vi "STM主程序（队列输入）-测试3.vi"() -> ()   [LabVIEW 2015]
uses:
  <vilib>/NI/STM/TCP/Write Meta Data (TCP Ref).vi
  <vilib>/NI/STM/NI STM.lvlib
  <vilib>/NI/STM/SubVIs/MetaDataElement.ctl
  <vilib>/NI/STM/TCP/Get Connection Reference (TCP).vi
  <vilib>/NI/STM/TCP/TCP Read Options.ctl
  <vilib>/NI/STM/TCP/Read Message (TCP).vi
  <vilib>/NI/STM/TCP/Write Message (TCP).vi
panel:
  in  "阈值等级":i32=4
  in  "Stop (F)":bool
  in  "关闭程序":bool
  out "触发":bool
  in  "?":bool
  out "自动后退":bool
  in  "?":bool
  out "自动前进":bool
  in  "?":bool
  out "步进距离":u16
  out "error  out":errorcluster
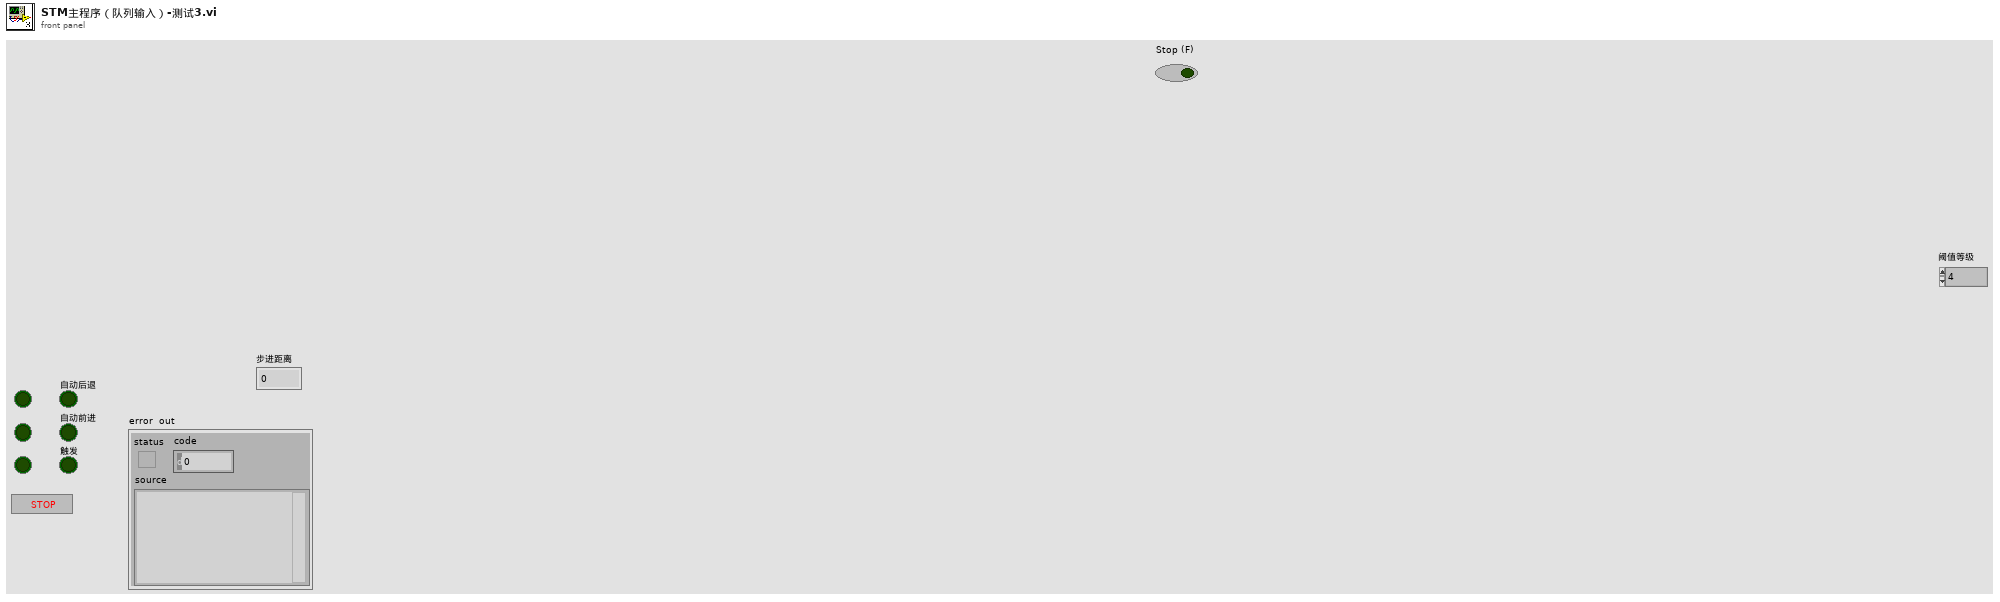
[diagram p1: front panel]
types:
  T1 = typedef "NI STM.lvlib/MetaDataElement.ctl" = string
  T2 = typedef "NI STM.lvlib/TCP Connection Info.ctl" = cluster{"connection ID":refnum<k5>, "meta data":T1[]}
  T3 = cluster{"图像数据":refnum<queue>, "队列输出":refnum<queue>}
  T4 = typedef "IMAQ Image.ctl" = refnum<image>
  T5 = cluster{"滤波":T4, "边缘检测":T4, "untitled":T4, "3D view":T4, "灰度图像":T4}
  T6 = cluster{"周长":dbl, "面积":dbl, "3D":u8[], "灰度图像":T4, "3D view":T4, "滤波":T4, "边缘检测":T4, "3D图像":T4, "质心坐标X":sgl, "质心坐标Y":sgl, "第一点y值，x=0":dbl, "第二点y值，x=639":dbl, "第一点x值，y=0":dbl, "第二点x值，y=479":dbl, "短轴半径um":dbl, "长轴半径um":dbl, "长轴长度":dbl, "短轴长度":dbl, "短轴原曲线":dbl[], "长轴拟合":dbl[], "纵轴拟合":dbl[], "横轴拟合":dbl[], "长轴原曲线":dbl[], "纵轴原曲线":dbl[], "横轴原曲线":dbl[], "短轴拟合":dbl[], "位置":dbl, "触发":bool, "初始化后退":bool, "初始化前进":bool}
  T7 = typedef "NI STM.lvlib/TCP Read Options.ctl" = cluster{"ignore timeout error":bool, "timeout ms (1000)":i32}
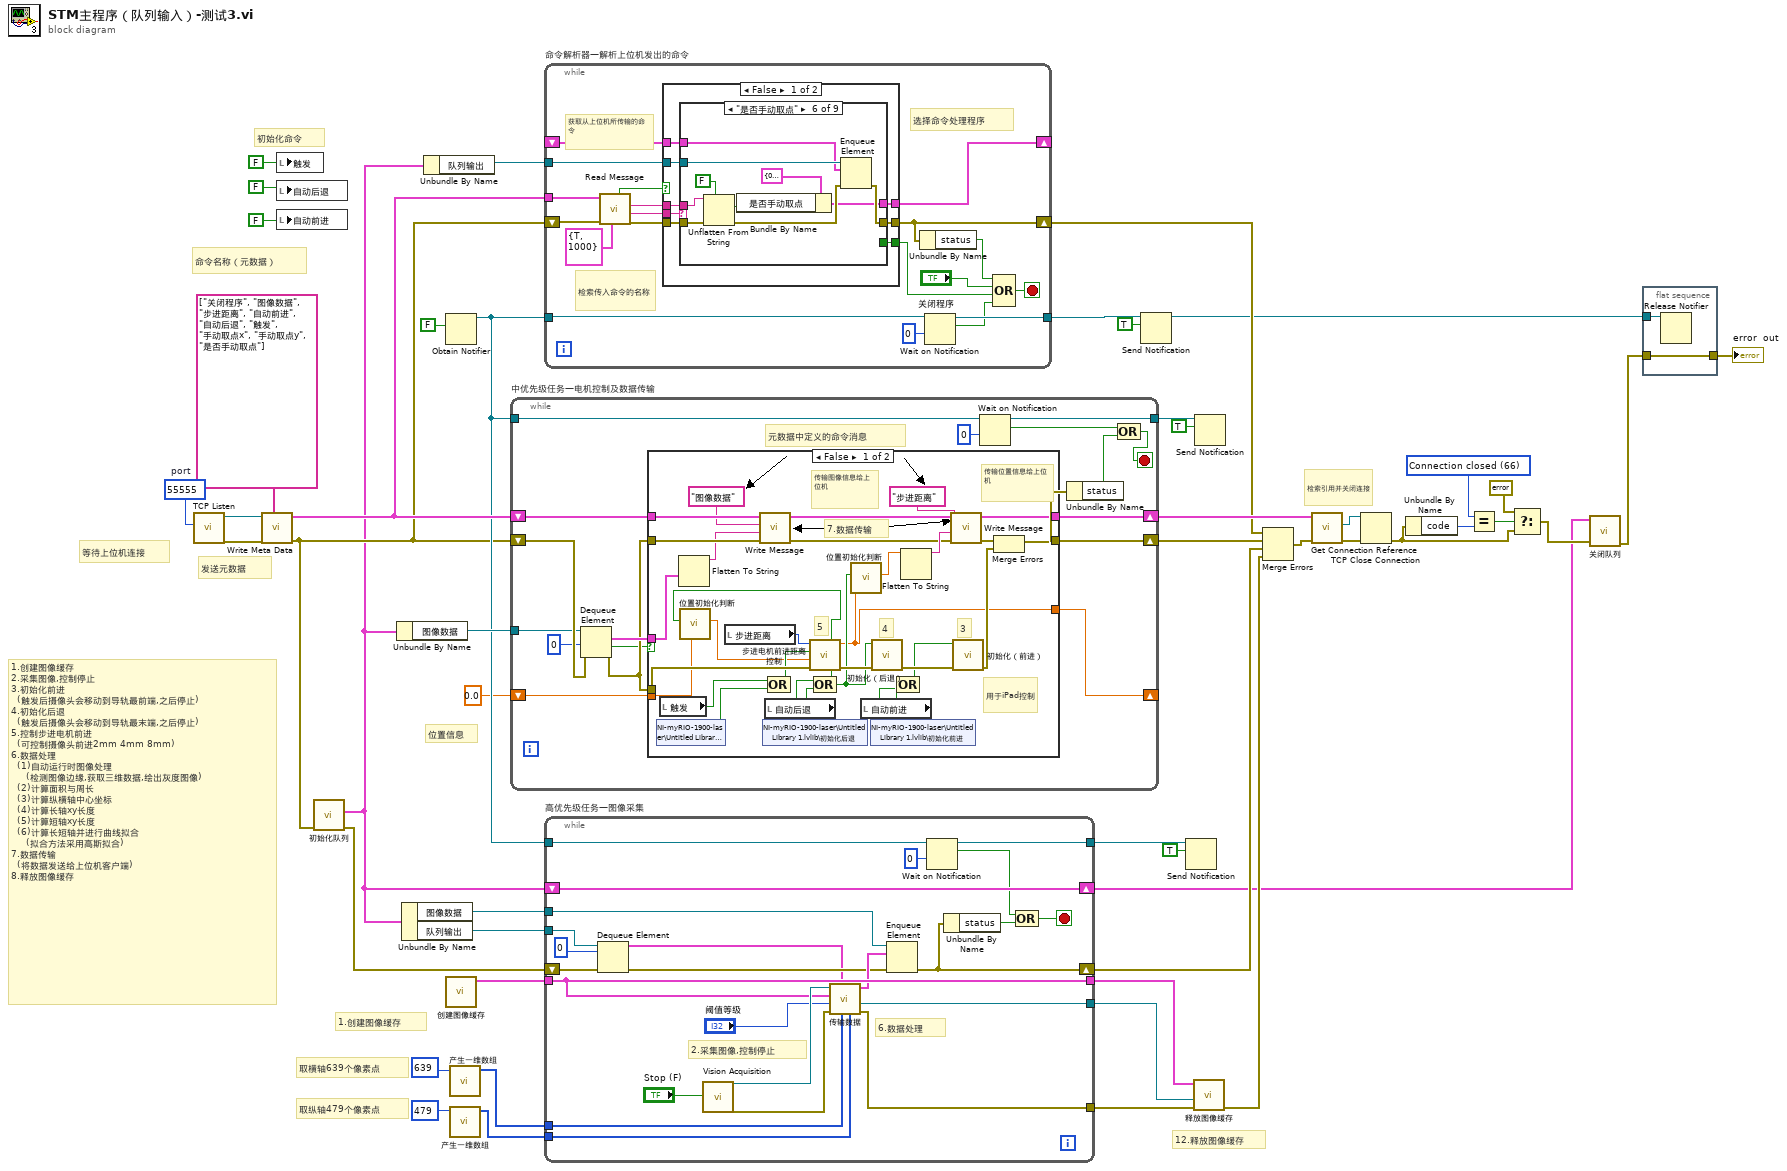
[diagram p0: block diagram]
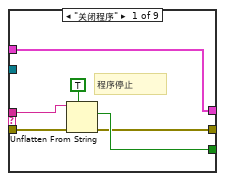
[diagram p3: hidden frame]
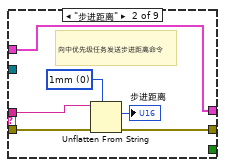
[diagram p4: hidden frame]
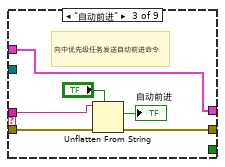
[diagram p5: hidden frame]
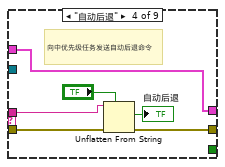
[diagram p6: hidden frame]
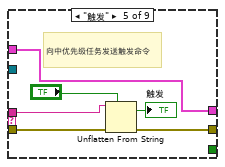
[diagram p7: hidden frame]
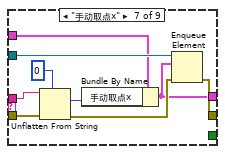
[diagram p8: hidden frame]
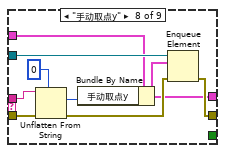
[diagram p9: hidden frame]
diagram:
  w24 = 66 items=["No Error", "Argument Error", "Memory Full", "Out of Zone", "End of File", "File Already Open", "Generic File IO Error", "File Not Found", "File Permission Error", "Disk Full", "Duplicate Path", "Too Many Files Open", "Not Enabled", "Resource File Not Found", "Cannot Add Resource", "Resource Not Found", "Image Not Found", "Image Memory Error", "Pen Does Not Exist", "Config Bad Type", "Config Token Not Found", "Config Parse Error", "Config Memory Error", "Bad External Code Format", "Bad External Code Offset", "External Code Not Present", "Null Window", "Destroy Window Mixup", "Null Menu", "Print Aborted", "Bad Print Record", "Print Driver Error", "Windows Error During Print", "Memory Error During Print", "Print Dialog Error", "Generic Print Error", "Invalid Device Refnum", "Device Not Found", "Device Parameter Error", "Device Unit Error", "Can't Open Device", "Device Call Aborted", "Generic Error", "Cancelled By User", "Object ID Too Low", "Object ID Too High", "Object Not In Heap", "Unknown Heap", "Bad DefProc ID", "DefProc Not In Table", "Message Out Of Range", "Null Method", "Unknown Message", "Manager Call Not Supported", "Bad address", "Connection In progress", "Connection timed out", "Connection is already in progress", "Network attribute not supported", "Network error", "Address in use", "System out of memory", "Connection aborted", "Connection refused", "Connection is not connected", "Connection is already connected", "Connection closed", "Initialize error (interapplication manager)", "Bad occurrence", "Wait on unbound occurrence handler", "Occurrence queue overflow", "Bad path", "Semaphore not signaled", "Unrecognized type (interapplication manager)"] ("1st Error to Convert")
  w50 = u16 55555  # port
  # "位置信息"
  # "初始化命令"
  # "等待上位机连接"
  # "发送元数据"
  # "检索引用并关闭连接"
  # "命令名称（元数据）"
  # "1.创建图像缓存"
  # "1.创建图像缓存\n2.采集图像,控制停止\n3.初始化前进\n  (触发后摄像头会移动到导轨最前端,之后停止)\n4.初始化后退\n  (触发后摄像头会移动到导轨最末端,之后停止)\n5.控制步进电机前进\n  (可控制摄像头前进2mm 4mm 8mm)\n6.数据处理\n  (1)自动运行时图像处理\n     (检测图像边缘,获取三维数据,绘出灰度图像)\n  (2)计算面积与周长\n  (3)计算纵横轴中心坐标\n  (4)计算长轴xy长度\n  (5)计算短轴xy长度\n  (6)计算长短轴并进行曲线拟合\n     (拟合方法采用高斯拟合) \n7.数据传输 \n  (将数据发送给上位机客户端) \n8.释放图像缓存"
  # "取纵轴479个像素点"
  # "取横轴639个像素点"
  # "12.释放图像缓存"
  n1 = call <vilib>:"TCP Listen.vi"("port"=w50) -> ("error out"=w48:errorcluster, "connection ID"=w49:refnum<k5>)  [unwired: 3 in, 6 out]
  n2 = call-poly "Write Meta Data.vi"("meta data"=T1[] ["关闭程序", "图像数据", "步进距离", "自动前进", "自动后退", "触发", "手动取点x", "手动取点y", "是否手动取点"] ("Meta data"), "error in"=w48, "connection ID"=w49) -> ("error out"=w21:errorcluster, "connection info out"=w47:T2)  [unwired: 2 in, 5 out]
  n3 = local write "触发"(FALSE) -> ()
  n4 = local write "自动后退"(FALSE) -> ()
  n5 = local write "自动前进"(FALSE) -> ()
  n6 = call "初始化队列.vi"("error in (no error)"=w21) -> ("error out"=w20:errorcluster, "输出簇"=w3:T3)  [unwired: 9 in]
  n7 = Unbundle By Name(w3) -> ("图像数据"=w46:refnum<queue>)
  n8 = Unbundle By Name(w3) -> ("图像数据"=w45:refnum<queue>, "队列输出"=w1:refnum<queue>)
  n9 = Unbundle By Name(w3) -> ("队列输出"=w2:refnum<queue>)
  n10 = Obtain Notifier(notification data type=FALSE) -> (notifier out=w31:refnum<notifier>)  [unwired: 3 in, 2 out]
  n11 = call "创建图像缓存.vi"() -> ("簇"=w19:T5)  [unwired: 11 in]
  n12 = call "产生一维数组.vi"("Numeric"=639) -> ("Array"=w10:i32[])  [unwired: 10 in]
  n13 = call "产生一维数组.vi"("Numeric"=479) -> ("Array"=w9:i32[])  [unwired: 10 in]
  n14 = while "中优先级任务—电机控制及数据传输" {
    tunnel: w46 -> [w58]
    shift-right: [w60] -> w41
    shift-left: w21 -> [w64]
    shift-right: [w66] -> w44
    shift-left: w47 -> [w67]
    tunnel: w31 -> [w61]
    tunnel: [w59] -> w32
    shift-right: [w56] -> _
    shift-left: 0.0 ("x") -> [w57]
    stop <- w51 stop-if-true
    # "元数据中定义的命令消息"
    n15 = Dequeue Element(queue=w58, timeout in ms (-1)=0, error in (no error)=w64) -> (element=w65:T6, timed out?=w54:bool, error out=w55:errorcluster)  [unwired: 1 out]
    n16 = case shown="False" w54 {
      tunnel: w67 -> [w97 w100]
      tunnel: w55 -> [w96 w99]
      tunnel: [w89 w100] -> w66
      tunnel: [w83 w99] -> w60
      tunnel: w65 -> [w81 _]
      tunnel: w57 -> [w72 w98]
      tunnel: [w69 w98] -> w56
      tunnel: w55 -> [w82 _]
      frame False {
        # "传输图像信息给上位机"
        # "用于iPad控制"
        # "传输位置信息给上位机"
        # "7.数据传输"
        # "3"
        # "4"
        # "5"
        n17 = shared-variable "NI-myRIO-1900-laser\\Untitled Library 1.lvlib\\触发"() -> (w79:bool)  [unwired: 1 in, 1 out]
        n18 = local read "触发"() -> (w80:bool)
        n19 = Flatten To String(anything=w81) -> (data string=w94:string)  [unwired: 1 in, 4 out]
        n20 = local read "步进距离"() -> (w88:u16)
        n21 = call-poly "Write Message.vi"("error in"=w96, "data"=w94, "name"="图像数据" ("Name"), "connection info in"=w97) -> ("error out"=w90:errorcluster, "connection info out"=w91:T2)  [unwired: 1 in, 5 out]
        n22 = shared-variable "NI-myRIO-1900-laser\\Untitled Library 1.lvlib\\初始化后退"() -> (w76:bool)  [unwired: 1 in, 1 out]
        n23 = local read "自动后退"() -> (w77:bool)
        n24 = Compound Arithmetic op=OR(w80, w79) -> (w78:bool)
        n25 = Compound Arithmetic op=OR(w77, w76) -> (w70:bool)
        n26 = call "位置初始化判断.vi"("位置初始化"=w72, "是否后退"=w70) -> ("位置判断"=w71:dbl)  [unwired: 9 in]
        n27 = call "步进电机前进距离控制.vi"("error in"=w82, "初始化位置"=w71, "触发"=w78, "枚举"=w88) -> ("error out"=w87:errorcluster, "位置"=w69:dbl)  [unwired: 6 in]
        n28 = call "位置初始化判断.vi"("位置初始化"=w69, "是否后退"=w70) -> ("位置判断"=w68:dbl)  [unwired: 9 in]
        n29 = local read "自动前进"() -> (w75:bool)
        n30 = shared-variable "NI-myRIO-1900-laser\\Untitled Library 1.lvlib\\初始化前进"() -> (w74:bool)  [unwired: 1 in, 1 out]
        n31 = call "初始化（后退）.vi"("error in"=w87, "初始化"=w70) -> ("error out"=w86:errorcluster)  [unwired: 9 in]
        n32 = Compound Arithmetic op=OR(w75, w74) -> (w73:bool)
        n33 = Flatten To String(anything=w68) -> (data string=w93:string)  [unwired: 1 in, 4 out]
        n34 = call-poly "Write Message.vi"("error in"=w90, "data"=w93, "name"="步进距离" ("Name"), "connection info in"=w91) -> ("error out"=w85:errorcluster, "connection info out"=w89:T2)  [unwired: 1 in, 5 out]
        n35 = call "初始化（前进）.vi"("error in"=w86, "初始化"=w73) -> ("error out"=w84:errorcluster)  [unwired: 9 in]
        n36 = Merge Errors(w85, w84) -> (w83:errorcluster)
      }
      frame True {
      }
    }
    n37 = Wait on Notification(notifier=w61, timeout in ms (-1)=0) -> (notifier out=w59:refnum<notifier>, notification=w53:bool)  [unwired: 2 in, 2 out]
    n38 = Unbundle By Name(w60) -> ("status"=w52:bool)
    n39 = Compound Arithmetic op=OR(w53, w52) -> (w51:bool)
  }
  n40 = while "命令解析器—解析上位机发出的命令" {
    tunnel: w47 -> [w119]
    shift-right: [w110] -> w39
    shift-left: w21 -> [w118]
    tunnel: w31 -> [w112]
    tunnel: [w106] -> w35
    tunnel: w2 -> [w103]
    shift-right: [w102] -> _
    shift-left: _ -> [w101]
    stop <- w107 stop-if-true
    # "选择命令处理程序"
    # "检索传入命令的名称"
    # "获取从上位机所传输的命令"
    n41 = call-poly <vilib>:"Read Message.vi"("options"=T7 {"ignore timeout error"=TRUE, "timeout ms (1000)"=1000} ("Options"), "error in"=w118, "connection info in"=w119) -> ("error out"=w114:errorcluster, "name"=w117:T1, "data string"=w116:string, "timed out?"=w115:bool)  [unwired: 2 in, 3 out]
    n42 = case shown="False" w115 {
      tunnel: w117 -> [w122 _]
      tunnel: w116 -> [w127 _]
      tunnel: w114 -> [w126 w189]
      tunnel: [w125 w189] -> w110
      tunnel: [w124 _] -> w104
      tunnel: w103 -> [w123 _]
      tunnel: [w121 w188] -> w102
      tunnel: w101 -> [w120 w188]
      frame False {
        n43 = case shown="\"是否手动取点\"" w122 {
          tunnel: w127 -> [w132 w136 w144 w150 w156 w164 w172 w185 _]
          tunnel: w126 -> [w131 w139 w145 w151 w157 w163 w173 w184 w187]
          tunnel: [w129 w138 w143 w149 w155 w162 w170 w179 w187] -> w125
          tunnel: [w130 _ _ _ _ _ _ _ _] -> w124
          tunnel: w123 -> [_ _ _ _ _ w161 w171 w183 _]
          tunnel: [w128 w134 w140 w146 w152 w159 w168 w177 w186] -> w121
          tunnel: w120 -> [w128 w134 w140 w146 w152 w158 w169 w178 w186]
          frame "关闭程序" {
            # "程序停止"
            n44 = Unflatten From String(type=TRUE, binary string=w132, error in (no error)=w131) -> (value=w130:bool, error out=w129:errorcluster)  [unwired: 1 in, 2 out]
          }
          frame "步进距离" {
            w137 = u16 0 items=["1mm", "2mm", "4mm", "8mm"] ("步进距离")
            # "向中优先级任务发送步进距离命令"
            n45 = Unflatten From String(type=w137, binary string=w136, error in (no error)=w139) -> (value=→"步进距离":u16, error out=w138:errorcluster)  [unwired: 1 in, 2 out]
          }
          frame "自动前进" {
            # "向中优先级任务发送自动前进命令"
            n46 = Unflatten From String(type="?", binary string=w144, error in (no error)=w145) -> (value=→"自动前进":bool, error out=w143:errorcluster)  [unwired: 1 in, 2 out]
          }
          frame "自动后退" {
            # "向中优先级任务发送自动后退命令"
            n47 = Unflatten From String(type="?", binary string=w150, error in (no error)=w151) -> (value=→"自动后退":bool, error out=w149:errorcluster)  [unwired: 1 in, 2 out]
          }
          frame "触发" {
            # "向中优先级任务发送触发命令"
            n48 = Unflatten From String(type="?", binary string=w156, error in (no error)=w157) -> (value=→"触发":bool, error out=w155:errorcluster)  [unwired: 1 in, 2 out]
          }
          frame "是否手动取点" {
            n49 = Unflatten From String(type=FALSE, binary string=w164, error in (no error)=w163) -> (value=w167:bool, error out=w165:errorcluster)  [unwired: 1 in, 2 out]
            n50 = Bundle By Name(cluster=cluster{"手动取点y":i32, "手动取点x":i32, "是否手动取点":bool} {"手动取点y"=0, "手动取点x"=0, "是否手动取点"=FALSE} ("手动取点"), "是否手动取点"=w167) -> (w159:cluster{"手动取点y":i32, "手动取点x":i32, "是否手动取点":bool})
            n51 = Enqueue Element(queue=w161, element=w158, error in (no error)=w165) -> (error out=w162:errorcluster)  [unwired: 3 out]
          }
          frame "手动取点x" {
            n52 = Unflatten From String(type=0 ("新值"), binary string=w172, error in (no error)=w173) -> (value=w176:i32, error out=w174:errorcluster)  [unwired: 1 in, 2 out]
            n53 = Bundle By Name(cluster=w169, "手动取点x"=w176) -> (w168:cluster{"手动取点y":i32, "手动取点x":i32, "是否手动取点":bool})
            n54 = Enqueue Element(queue=w171, element=w168, error in (no error)=w174) -> (error out=w170:errorcluster)  [unwired: 3 out]
          }
          frame "手动取点y" {
            n55 = Unflatten From String(type=0 ("新值"), binary string=w185, error in (no error)=w184) -> (value=w182:i32, error out=w180:errorcluster)  [unwired: 1 in, 2 out]
            n56 = Bundle By Name(cluster=w178, "手动取点y"=w182) -> (w177:cluster{"手动取点y":i32, "手动取点x":i32, "是否手动取点":bool})
            n57 = Enqueue Element(queue=w183, element=w177, error in (no error)=w180) -> (error out=w179:errorcluster)  [unwired: 3 out]
          }
          frame Default {
          }
        }
      }
      frame True {
      }
    }
    n58 = Unbundle By Name(w110) -> ("status"=w109:bool)
    n59 = Wait on Notification(notifier=w112, timeout in ms (-1)=0) -> (notifier out=w106:refnum<notifier>, notification=w105:bool)  [unwired: 2 in, 2 out]
    n60 = Compound Arithmetic op=OR(w109, "关闭程序", w104, w105) -> (w107:bool)
  }
  n61 = while "高优先级任务—图像采集" {
    tunnel: w45 -> [w213]
    shift-right: [w209] -> w40
    shift-left: w20 -> [w192]
    shift-right: [w212] -> w7
    shift-left: w3 -> [w212]
    tunnel: w31 -> [w210]
    tunnel: [w205] -> w29
    tunnel: [w200] -> w18
    tunnel: [w199] -> w17
    tunnel: w10 -> [w197]
    tunnel: w9 -> [w196]
    tunnel: w19 -> [w198]
    tunnel: [w198] -> w16
    tunnel: w1 -> [w193]
    stop <- w206 stop-if-true
    # "6.数据处理"
    # "2.采集图像,控制停止"
    n62 = Dequeue Element(queue=w193, timeout in ms (-1)=0, error in (no error)=w192) -> (element=w190:cluster{"手动取点y":i32, "手动取点x":i32, "是否手动取点":bool}, error out=w191:errorcluster)  [unwired: 2 out]
    n63 = call "Vision Acquisition"("Stop (F)"="Stop (F)") -> ("Image Out"=w204:T4, "error out"=w203:errorcluster)  [unwired: 22 in, 3 out]
    n64 = call "传输数据.vi"("纵轴数组"=w196, "横纵数组"=w197, "输出簇"=w190, "error in (no error)"=w203, "阈值等级"="阈值等级", "配置缓存"=w198, "Image Src"=w204) -> ("error out"=w200:errorcluster, "灰度图像"=w199:T4, "已采集数据"=w195:T6)  [unwired: 2 in]
    n65 = Enqueue Element(queue=w213, element=w195, error in (no error)=w191) -> (error out=w209:errorcluster)  [unwired: 3 out]
    n66 = Wait on Notification(notifier=w210, timeout in ms (-1)=0) -> (notifier out=w205:refnum<notifier>, notification=w207:bool)  [unwired: 2 in, 2 out]
    n67 = Unbundle By Name(w209) -> ("status"=w208:bool)
    n68 = Compound Arithmetic op=OR(w207, w208) -> (w206:bool)
  }
  n69 = Send Notification(notification=TRUE, notifier=w35) -> (notifier out=w28:refnum<notifier>)  [unwired: 1 in, 1 out]
  n70 = Send Notification(notification=TRUE, notifier=w29) -> ()  [unwired: 1 in, 2 out]
  n71 = call "释放图像缓存.vi"("错误输入（无错误）"=w18, "灰度图像"=w17, "缓存数据"=w16) -> ("错误输出"=w15:errorcluster)  [unwired: 8 in]
  n72 = Send Notification(notification=TRUE, notifier=w32) -> ()  [unwired: 1 in, 2 out]
  n73 = Merge Errors(w39, w41, w40, w15) -> (w38:errorcluster)
  n74 = call-poly <vilib>:"Get Connection Reference.vi"("error in"=w38, "connection info in"=w44) -> ("error out"=w42:errorcluster, "connection ID out"=w43:refnum<k5>)  [unwired: 8 out]
  n75 = TCP Close Connection(connection ID=w43, error in (no error)=w42) -> (error out=w23:errorcluster)  [unwired: 2 out]
  n76 = Unbundle By Name(w23) -> ("code"=w26:i32)
  n77 = Equal?(x=w24, y=w26) -> (x = y?=w25:bool)
  n78 = Select(t=errorcluster {"status"=FALSE, "code"=0, "source"=""}, s=w25, f=w23) -> (s? t:f=w14:errorcluster)
  n79 = call "关闭队列.vi"("error in (no error)"=w14, "输出簇"=w7) -> ("error out"=w13:errorcluster)  [unwired: 9 in]
  n80 = flat-sequence {
    tunnel: w28 -> [w215]
    tunnel: w13 -> [w214]
    tunnel: [w214] -> w27
    frame #0 {
      n81 = Release Notifier(notifier=w215) -> ()  [unwired: 2 in, 3 out]
    }
  }
  "error  out" <- w27
